vi "niRFUtil MT Generate Filter Coefficients.vi"(0 "pulse shaping filter (none)":T3(ring), 1 "modulation type":T2(ring), 5 "pulse shaping samples per symbol (16)":i32=16, 7 "matched samples per symbol (16)":i32=16, 9 "filter parameter":dbl=0.5 format="%.2f", 11 "error in (no error)":errorcluster, 12 "filter length (symbols)":i32=8) -> (4 "pulse shaping filter coefficients":T1 min=0 max=127 format="%.2f", 6 "matched filter coefficients":T1 min=0 max=127 format="%.2f", 15 "error out":errorcluster)   [LabVIEW 2015, in "niRFUtil.lvlib"]
doc: "Calculates filter coefficients for pulse-shaping and matched filters applied by the digital modulation VIs and demodulation VIs."
uses:
  niRFUtil.lvlib
  Includes/niRFUtil INC Real Array.ctl
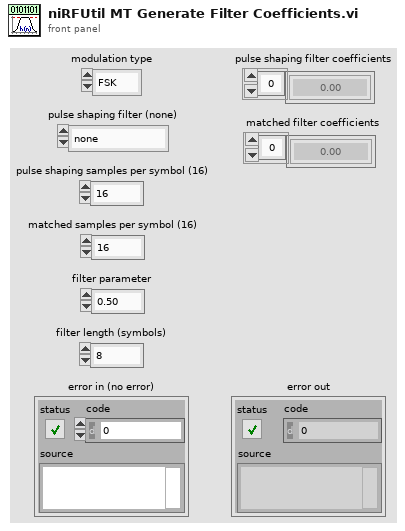
[diagram p1: front panel]
types:
  T1 = typedef "niRFUtil.lvlib/niRFUtil INC Real Array.ctl" = sgl[]
  T2 = enum16{"FSK", "PSK", "QAM", "MSK", "PAM", "ASK", "CPM"}
  T3 = enum16{"none", "Raised Cosine", "Root Raised Cos", "Gaussian"}
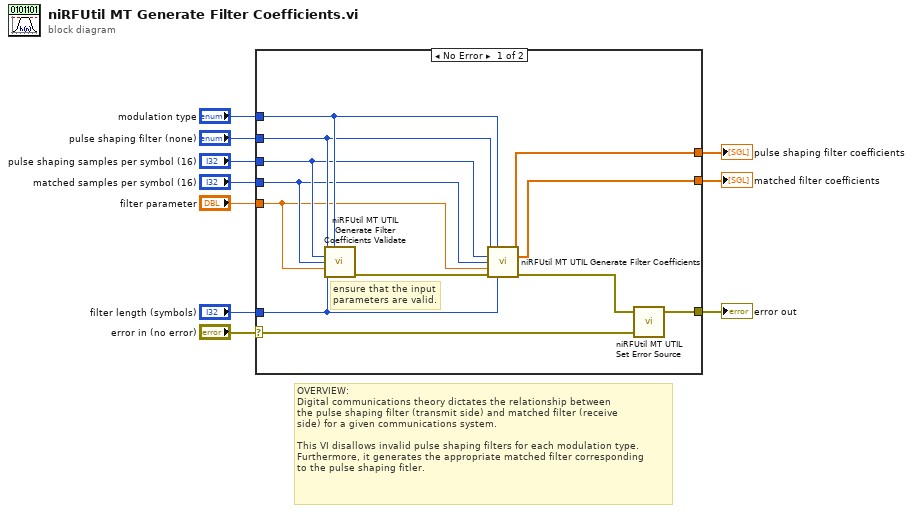
[diagram p0: block diagram]
diagram:
  # "OVERVIEW:\nDigital communications theory dictates the relationship between\nthe pulse shaping filter (transmit side) and matched filter (receive\nside) for a given communications system.\n\nThis VI disallows invalid pulse shaping filters for each modulation type.\nFurthermore, it generates the appropriate matched filter corresponding\nto the pulse shaping fitler."
  n1 = case shown="No Error" "error in (no error)" {
    selector: "error in (no error)" -> [w19 w23]
    tunnel: "pulse shaping filter (none)" -> [w16 _]
    tunnel: "pulse shaping samples per symbol (16)" -> [w15 _]
    tunnel: "filter length (symbols)" -> [w18 _]
    tunnel: "filter parameter" -> [w13 _]
    tunnel: [w21 w23] -> w5
    tunnel: [w12 _] -> w1
    tunnel: "modulation type" -> [w17 _]
    tunnel: "matched samples per symbol (16)" -> [w14 _]
    tunnel: [w11 _] -> w2
    frame No Error {
      # "ensure that the input parameters are valid."
      n2 = call "niRFUtil MT UTIL Generate Filter Coefficients Validate.vi"("System Filter Characteristic (none)"=w16, "Modulation Type"=w17, "Modulation Samples Per Symbol (16)"=w15, "Demodulation Samples Per Symbol (16)"=w14, "Filter Parameter"=w13, "Filter Length (3)"=w18) -> ("error out"=w22:errorcluster)  [unwired: 9 out]
      n3 = call "niRFUtil MT UTIL Generate Filter Coefficients.vi"("System Filter Characteristic (none)"=w16, "Modulation Type"=w17, "Modulation Samples Per Symbol (16)"=w15, "Demodulation Samples Per Symbol (16)"=w14, "Filter Parameter"=w13, "error in (no error)"=w22, "Filter Length (3)"=w18) -> ("Pulse Shaping Filter Coefficients"=w12:T1, "Matched Filter Coefficients"=w11:T1, "error out"=w20:errorcluster)  [unwired: 6 out]
      n4 = call "niRFUtil MT UTIL Set Error Source.vi"("initial error in (no error)"=w19, "final error in (no error)"=w20) -> ("error out"=w21:errorcluster)  [unwired: 3 in]
    }
    frame Error {
    }
  }
  "error out" <- w5
  "pulse shaping filter coefficients" <- w1
  "matched filter coefficients" <- w2
